vi "CSTK_BuildApplication_Manager_Post-Build Action.vi"(5 "Files Generated by Build":path[](array[path]) caption="通过生成创建的文件", 6 "Top Level/Always Included VIs":path[](array[path]) caption="顶层/始终包括VI", 7 "Destination Path":path caption="目标路径", 8 "error in (no error)":errorcluster caption="错误输入（无错误）", 9 "Target Name":string caption="终端名称", 10 "Build Specification Name":string caption="程序生成规范名称", 11 "Project Path":path caption="项目路径") -> (0 "error out":errorcluster caption="错误输出")   [LabVIEW 2015]
uses:
  CSTK_BuildApplication_Manager.lvlib
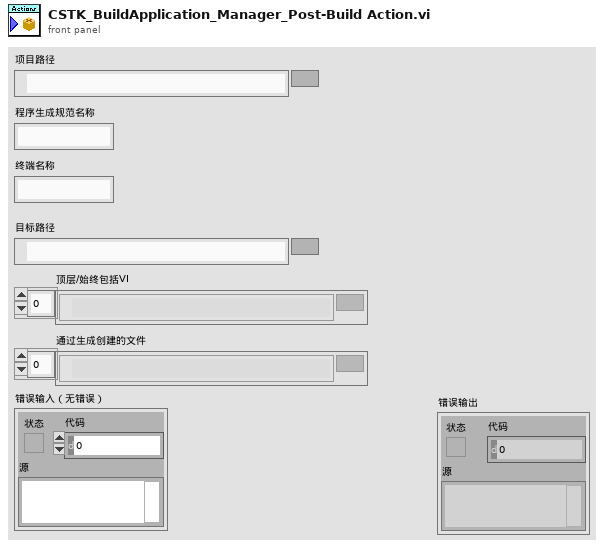
[diagram p1: front panel]
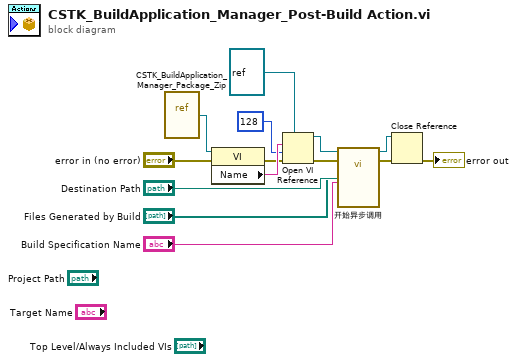
[diagram p0: block diagram]
diagram:
  n1 = vi-ref "CSTK_BuildApplication_Manager_Package_Zip.vi"() -> (w14:refnum<vi>)
  n2 = property class="VI"(reference=w14, error in="error in (no error)") -> (error out=w8:errorcluster, "Name"=w13:string)  [unwired: 1 out]
  n3 = Open VI Reference(type specifier VI Refnum (for type only)=refnum<vi> refnum ("类型说明符VI引用句柄（仅用于类型）"), vi path=w13, options=128 ("选项"), error in (no error)=w8) -> (vi reference=w10:refnum<vi>, error out=w9:errorcluster)  [unwired: 2 in]
  n4 = call-by-ref "开始异步调用"(reference=w10, error in=w9, "Files Generated by Build"="Files Generated by Build", "Destination Path"="Destination Path", "Build Specification Name"="Build Specification Name") -> (reference out=w3:refnum<vi>, error out=w2:errorcluster)  [unwired: 8 in, 1 out]
  n5 = Close Reference(reference=w3, error in (no error)=w2) -> (error out=→"error out":errorcluster)
